vi "Channel Initialize.vi"(0 "Item Ref in":T2 format="%.0x", 7 "error in (no error)":errorcluster, 8 "Starting Address Ref in":refnum<vi>) -> (16 "Radix":T1, 17 "Sub-Index (Bool)":u16, 18 "Registers":i32, 19 "input?":bool, 20 "Channel Ref out":T2 format="%.0x", 21 "Name":string, 22 "Description":string, 23 "Starting Address":u16, 24 "DataType":T3, 25 "Valid?":bool, 26 "Status Message":string, 27 "error out":errorcluster)   [LabVIEW 2015, in "Modbus Master System Explorer.lvlib"]
uses:
  Modbus Master System Explorer.lvlib
  Shared/Controls/Data Model/DataType.ctl
  <vilib>/NI Veristand/Custom Device API/Custom Device Item Ref.ctl
  Radix.ctl
  <vilib>/NI VeriStand/Custom Device API/Custom Device API.lvlib
  Shared/Modbus Master Shared.lvlib
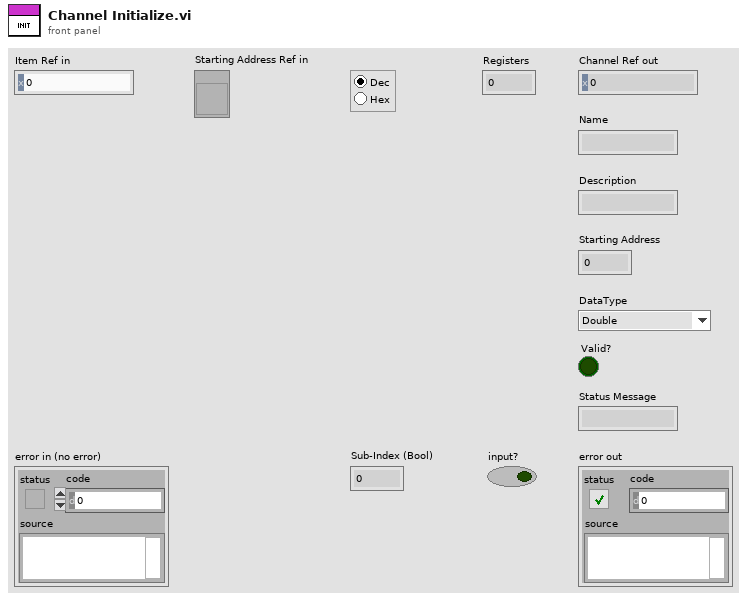
[diagram p1: front panel]
types:
  T1 = typedef "Modbus Master System Explorer.lvlib/Radix.ctl" = enum32{"Decimal", "Hexidecimal"}
  T2 = typedef "Custom Device API.lvlib/Custom Device Item Ref.ctl" = u64
  T3 = typedef "Modbus Master Shared.lvlib/DataType.ctl" = enum16{"Double", "Single", "I64", "I32", "I16", "I8", "U64", "U32", "U16", "U8", "Boolean"}
  T4 = typedef "Custom Device API.lvlib/Custom Device Item Info.ctl" = cluster{"Name":string, "Is Channel":bool, "GUID":string, "Is Waveform":bool}
  T5 = typedef "Modbus Master Shared.lvlib/Mapping.ctl" = cluster{"DataType":T3, "Starting Address":u16, "Sub-Index (Bool)":u16, "VS Reference":T2}
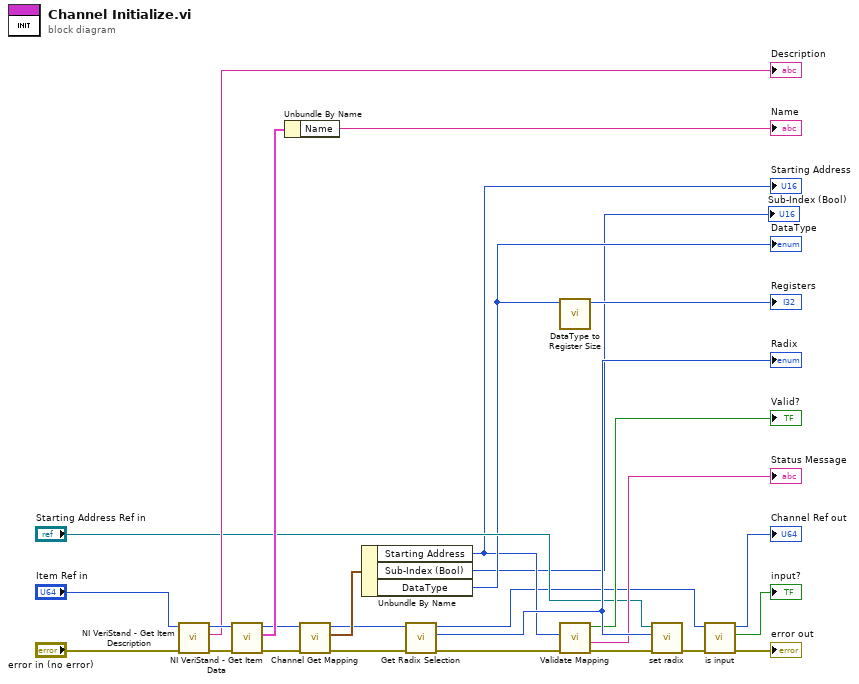
[diagram p0: block diagram]
diagram:
  n1 = call <vilib>:"NI VeriStand - Get Item Description.vi"("error in (no error)"="error in (no error)", "Item Ref in"="Item Ref in") -> ("error out"=w26:errorcluster, "Description"=→"Description":string, "Item Ref out"=w27:T2)  [unwired: 7 out]
  n2 = call <vilib>:"NI VeriStand - Get Item Data.vi"("error in (no error)"=w26, "Item Ref in"=w27) -> ("error out"=w23:errorcluster, "Item Info"=w25:T4, "Item Ref out"=w24:T2)  [unwired: 7 out]
  n3 = Unbundle By Name(w25) -> ("Name"=→"Name":string)
  n4 = call "Channel Get Mapping.vi"("error in (no error)"=w23, "Item Ref in"=w24) -> ("error out"=w20:errorcluster, "Mapping"=w22:T5, "Item Ref out"=w21:T2)  [unwired: 7 in]
  n5 = Unbundle By Name(w22) -> ("Starting Address"=w7:u16, "Sub-Index (Bool)"=→"Sub-Index (Bool)":u16, "DataType"=w8:T3)
  "Starting Address" <- w7
  "DataType" <- w8
  n6 = call "Get Radix Selection.vi"("error in (no error)"=w20, "Item Ref in"=w21) -> ("error out"=w19:errorcluster, "Radix"=w18:T1, "Item Ref out"=w4:T2)  [unwired: 7 in]
  "Radix" <- w18
  n7 = call "DataType to Register Size.vi"("DataType"=w8) -> ("Registers"=→"Registers":i32)  [unwired: 9 in, 1 out]
  n8 = call "Validate Mapping.vi"("error in (no error)"=w19, "Mapping"=w7) -> ("error out"=w17:errorcluster, "Status Message"=→"Status Message":string, "Valid?"=→"Valid?":bool)  [unwired: 7 in]
  n9 = call "set radix.vi"("error in (no error)"=w17, "Radix"=w18, "Digital in"="Starting Address Ref in") -> ("error out"=w6:errorcluster)  [unwired: 8 in]
  n10 = call "is input.vi"("error in (no error)"=w6, "Item Ref in"=w4) -> ("error out"=→"error out":errorcluster, "input?"=→"input?":bool, "Channel Ref out"=→"Channel Ref out":T2)  [unwired: 7 in]
